vi "Write Base Actor.vi"(10 "Base Actor":T1, 11 "Actor in":refnum<class "Actor.lvclass">) -> (3 "Actor out":refnum<class "Actor.lvclass">)   [LabVIEW 2020, in "jettl.lvlib" / "Actor.lvclass"]
uses:
  Actor.lvclass
  Msg/Msg.lvclass
  Msg Input/Msg Input.lvclass
  Msg Output/Msg Output.lvclass
  Unified Actor Lifetime.ctl
  jettl.lvlib
  Base Actor.ctl
  Unified Actor Relation.ctl
  Teller.ctl
  Msg.ctl
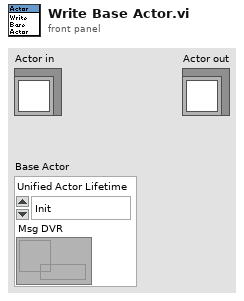
[diagram p1: front panel]
types:
  T1 = typedef "jettl.lvlib/Base Actor.ctl" = cluster{"Unified Actor Lifetime":T2, "Msg DVR":refnum<data-value>}
  T2 = typedef "jettl.lvlib/Unified Actor Lifetime.ctl" = enum16{"Init", "Spawn", "Setup", "Teardown Before Running", "Running", "Stop Called", "Stopping With Children", "Stopping Without Children", "Teardown After Running", "Stopped"}
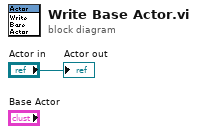
[diagram p0: block diagram]
diagram:
  "Actor out" <- "Actor in"
